vi "Write Test Case object to front panel control.vi"(8 "error in (no error)":errorcluster, 11 "LUnit Test Case In":refnum<class "LUnit Test Case.lvclass">) -> (0 "error out":errorcluster, 3 "LUnit Test Case Out":refnum<class "LUnit Test Case.lvclass">)   [LabVIEW 2020, in "LUnit Test Case.lvclass"]
uses:
  LUnit Test Case.lvclass
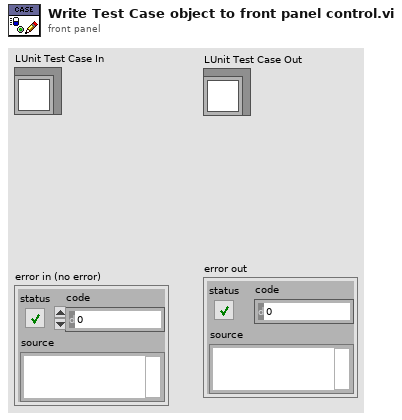
[diagram p1: front panel]
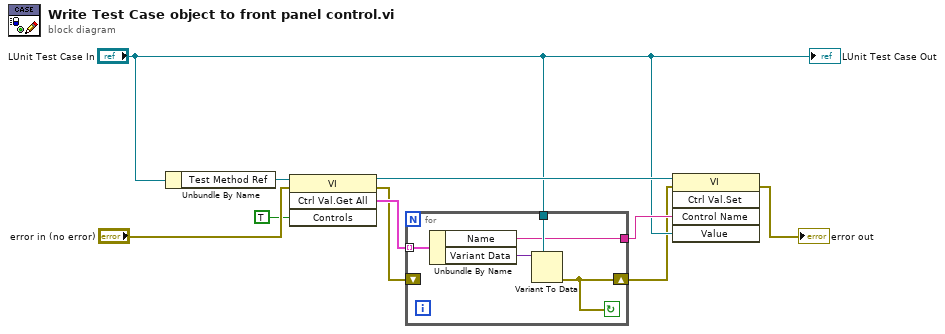
[diagram p0: block diagram]
diagram:
  n1 = Unbundle By Name("LUnit Test Case In") -> ("Test Method Ref"=w4:refnum<vi>)
  n2 = invoke on="Invoke Node" class="VI" method="Ctrl Val.Get All"(reference=w4, error in="error in (no error)", "Controls"=TRUE) -> (reference out=w6:refnum<vi>, error out=w2:errorcluster, "Get All Control Values Variant"=w8:cluster{"Name":string, "Variant Data":variant}[])  [unwired: 1 in, 1 out]
  n3 = for {
    tunnel: w8 -> [w15] mode=indexing
    tunnel: "LUnit Test Case In" -> [w13]
    tunnel: [w12] -> w9
    shift-right: [w11] -> w1
    shift-left: w2 -> [_]
    stop <- w11 continue-if-true
    n4 = Unbundle By Name(w15) -> ("Name"=w12:string, "Variant Data"=w14:variant)
    n5 = Variant To Data(type=w13, Variant=w14) -> (error out=w11:errorcluster)  [unwired: 1 in, 1 out]
  }
  n6 = invoke on="Invoke Node" class="VI" method="Ctrl Val.Set"(reference=w6, error in=w1, "Control Name"=w9, "Value"="LUnit Test Case In") -> (error out=→"error out":errorcluster)  [unwired: 1 in, 4 out]
  "LUnit Test Case Out" <- "LUnit Test Case In"
